vi "RTTouchVariables.vi"(8 "error in (no error)":errorcluster) -> (0 "error out":errorcluster)   [LabVIEW 2016]
uses:
  controls/MotorSetStates.ctl
  controls/MotorStates.ctl
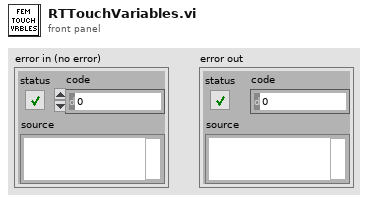
[diagram p1: front panel]
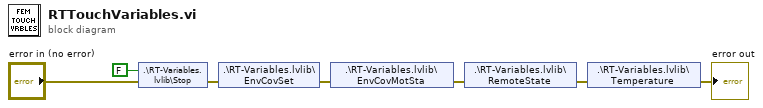
[diagram p0: block diagram]
diagram:
  n1 = shared-variable ".\\RT-Variables.lvlib\\Stop"(FALSE ("Stop"), error in="error in (no error)") -> (error out=w1:errorcluster)
  n2 = shared-variable ".\\RT-Variables.lvlib\\EnvCovSet"(error in=w1) -> (error out=w5:errorcluster)  [unwired: 1 out]
  n3 = shared-variable ".\\RT-Variables.lvlib\\EnvCovMotSta"(error in=w5) -> (error out=w6:errorcluster)  [unwired: 1 out]
  n4 = shared-variable ".\\RT-Variables.lvlib\\RemoteState"(error in=w6) -> (error out=w7:errorcluster)  [unwired: 1 out]
  n5 = shared-variable ".\\RT-Variables.lvlib\\Temperature"(error in=w7) -> (error out=→"error out":errorcluster)  [unwired: 1 out]
